vi "Test Get VIs in project excludes LV Root.vi"(8 "error in (no error)":errorcluster, 11 "Test Case In":refnum<class "Coverage Test.lvclass">) -> (0 "error out":errorcluster, 3 "Test Case Out":refnum<class "Coverage Test.lvclass">)   [LabVIEW 2020, in "LUnit Tests.lvlib" / "Coverage Test.lvclass"]
uses:
  Coverage Test.lvclass
  C:/Program Files (x86)/National Instruments/LabVIEW 2020/vi.lib/Astemes/LUnit/Test Case.lvclass
  source/Framework/Coverage Analyzer/Coverage Analyzer.lvclass
  <vilib>/Astemes/LUnit/Test Case.lvclass/Test Case.ctl
  <vilib>/Astemes/LUnit/LUnit Assertion Result.lvclass/LUnit Assertion Result.ctl
  <vilib>/Astemes/LUnit/LUnit Test Case Result.lvclass/LUnit Test Case Result.ctl
  <vilib>/Astemes/LUnit/LUnit Method Result.lvclass/LUnit Method Result.ctl
  01074fa8-ee8a-411d-bc8b-fc92c4f90959.vi
  <vilib>/Astemes/LUnit/Palette/Pass.vi
  <vilib>/Astemes/LUnit/Palette/Fail.vi
  <vilib>/Astemes/LUnit/Compare Variants.vi
  <vilib>/Astemes/LUnit/Describe Comparison.vi
  <vilib>/Astemes/LUnit/Set Assertion Type.vi
  <vilib>/Astemes/LUnit/Add test result.vi
  <vilib>/Astemes/LUnit/LUnit Write Passed.vi
  <vilib>/Astemes/LUnit/LUnit Write Message.vi
  <vilib>/Astemes/LUnit/LUnit Write Description.vi
  <vilib>/Astemes/LUnit/Variant to string.vi
  <vilib>/Astemes/LUnit/LUnit Write Assertion Type.vi
  <vilib>/Astemes/LUnit/LUnit Record Assertion Result.vi
  <vilib>/Astemes/LUnit/LUnit Aggregate Assertion Results.vi
  <vilib>/Astemes/LUnit/Assertion Result/LUnit Read Status.vi
  <vilib>/Astemes/LUnit/LUnit Read Message.vi
  <vilib>/Astemes/LUnit/LUnit Read Description.vi
  <vilib>/Astemes/LUnit/Method Result/LUnit Merge Status.vi
  <vilib>/Astemes/LUnit/LUnit Concatenate result strings.vi
  <vilib>/Utility/Data Type/Get Type Information.vi
  <vilib>/Utility/LVClass/Get LV Class Name.vi
  <vilib>/Astemes/LUnit/LUnit Assertion Result.lvclass
  Coverage Test.lvclass/Coverage Test.ctl
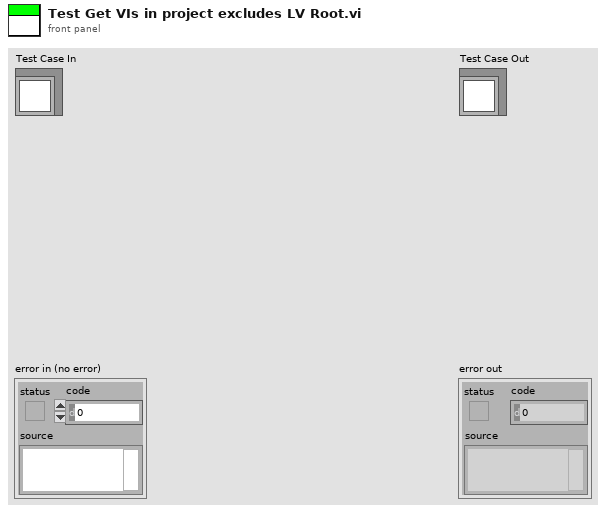
[diagram p1: front panel]
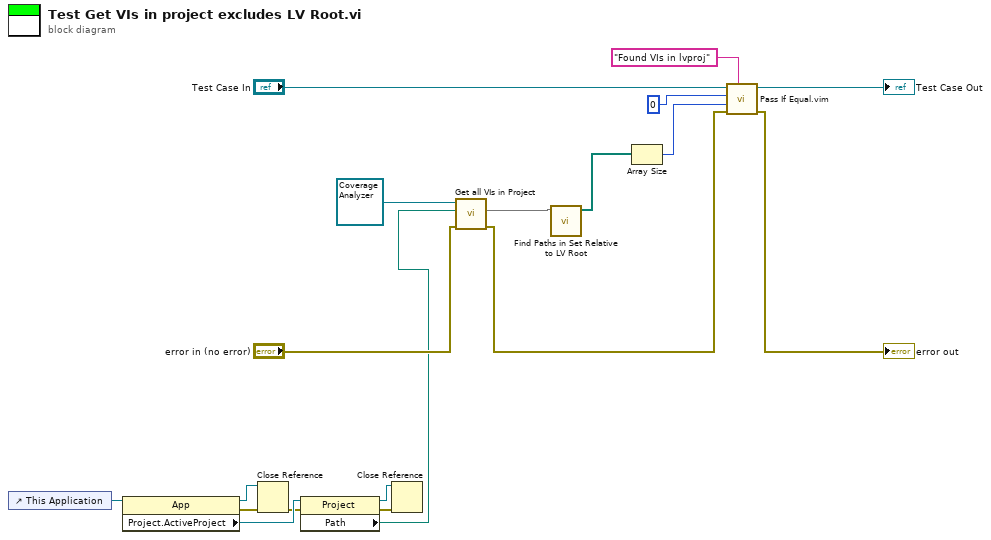
[diagram p0: block diagram]
diagram:
  n1 = control-ref of="This Application"() -> (w8:refnum<vi>)
  n2 = property class="App"(reference=w8) -> (reference out=w6:refnum<vi>, error out=w3:errorcluster, "Project.ActiveProject"=w7:refnum<vi>)  [unwired: 1 in]
  n3 = Close Reference(reference=w6, error in (no error)=w3) -> (error out=w2:errorcluster)
  n4 = property class="Project"(reference=w7, error in=w2) -> (reference out=w5:refnum<vi>, error out=w4:errorcluster, "Path"=w1:path)
  n5 = Close Reference(reference=w5, error in (no error)=w4) -> ()  [unwired: 1 out]
  n6 = call "Get all VIs in Project.vi"("error in (no error)"="error in (no error)", "Path"=w1, "Coverage Analyzer in"=refnum<class "Coverage Analyzer.lvclass"> refnum ("Coverage Analyzer.lvclass")) -> ("error out"=w9:errorcluster, "VIs"=w12:set{path})  [unwired: 6 in, 1 out]
  n7 = call "Find Paths in Set Relative to LV Root.vi"("VIs"=w12) -> ("Array"=w11:path[])  [unwired: 10 in]
  n8 = Array Size(array=w11) -> (size(s)=w15:i32)
  n9 = call "Pass If Equal.vim"("Description"="Found VIs in lvproj", "error in (no error)"=w9, "Actual"=w15, "Expected"=0 ("size(s)"), "LUnit Test Case In"="Test Case In") -> ("error out"=→"error out":errorcluster, "LUnit Test Case Out"=→"Test Case Out":refnum<class "Coverage Test.lvclass">)  [unwired: 5 in]
